vi "硬件定时参数设置.vi"(11 "硬件定时配置输入":T1) -> (3 "硬件定时配置输出":u32[](array[numeric]))   [LabVIEW 2012]
uses:
  u32-u8s.vi
  u16-u8s.vi
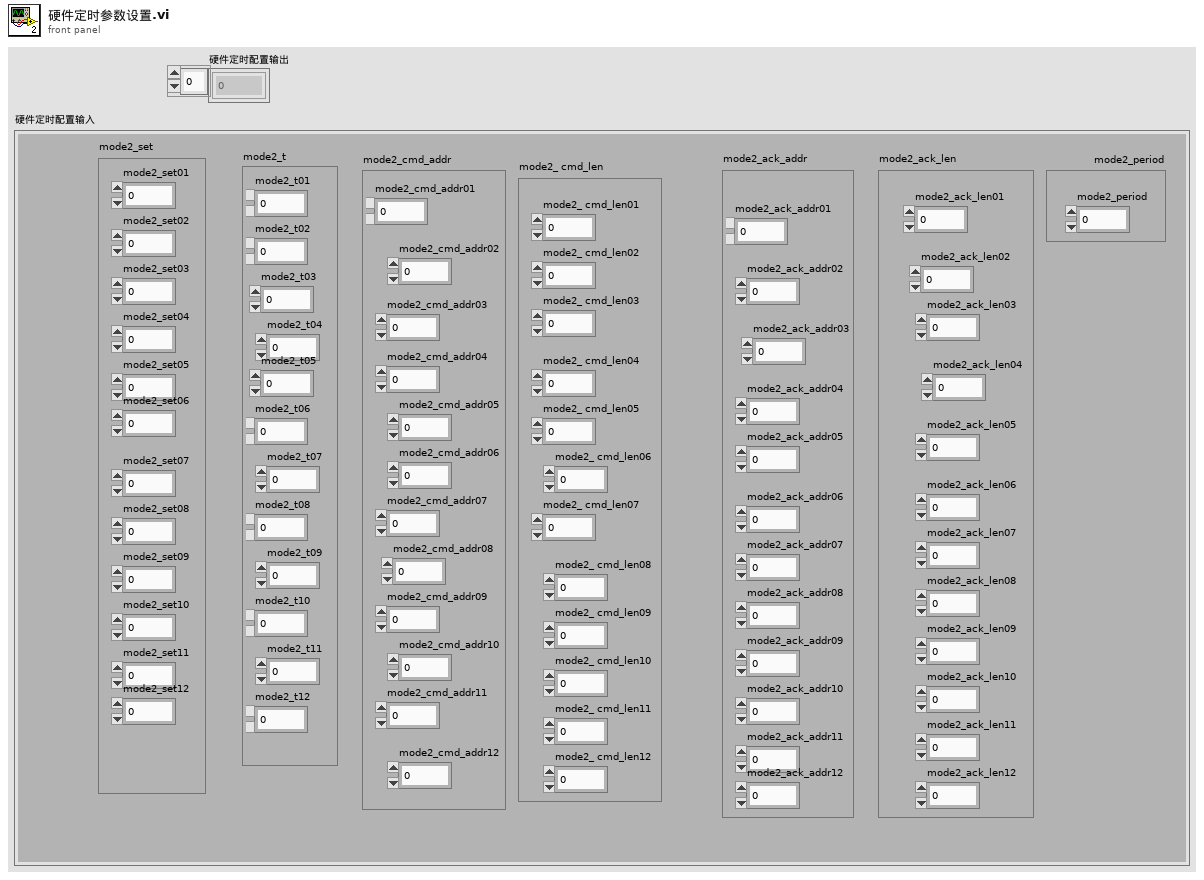
[diagram p1: front panel]
types:
  T1 = cluster{"mode2_set":cluster{"mode2_set01":u8, "mode2_set02":u8, "mode2_set03":u8, "mode2_set04":u8, "mode2_set05":u8, "mode2_set06":u8, "mode2_set07":u8, "mode2_set08":u8, "mode2_set09":u8, "mode2_set10":u8, "mode2_set11":u8, "mode2_set12":u8}, "mode2_t":cluster{"mode2_t01":u16, "mode2_t02":u16, "mode2_t03":u16, "mode2_t04":u16, "mode2_t05":u16, "mode2_t06":u16, "mode2_t07":u16, "mode2_t08":u16, "mode2_t09":u16, "mode2_t10":u16, "mode2_t11":u16, "mode2_t12":u16}, "mode2_cmd_addr":cluster{"mode2_cmd_addr01":u16, "mode2_cmd_addr02":u16, "mode2_cmd_addr03":u16, "mode2_cmd_addr04":u16, "mode2_cmd_addr05":u16, "mode2_cmd_addr06":u16, "mode2_cmd_addr07":u16, "mode2_cmd_addr08":u16, "mode2_cmd_addr09":u16, "mode2_cmd_addr10":u16, "mode2_cmd_addr11":u16, "mode2_cmd_addr12":u16}, "mode2_ cmd_len":cluster{"mode2_ cmd_len01":u16, "mode2_ cmd_len02":u16, "mode2_ cmd_len03":u16, "mode2_ cmd_len04":u16, "mode2_ cmd_len05":u16, "mode2_ cmd_len06":u16, "mode2_ cmd_len07":u16, "mode2_ cmd_len08":u16, "mode2_ cmd_len09":u16, "mode2_ cmd_len10":u16, "mode2_ cmd_len11":u16, "mode2_ cmd_len12":u16}, "mode2_ack_addr":cluster{"mode2_ack_addr01":u16, "mode2_ack_addr02":u16, "mode2_ack_addr03":u16, "mode2_ack_addr04":u16, "mode2_ack_addr05":u16, "mode2_ack_addr06":u16, "mode2_ack_addr07":u16, "mode2_ack_addr08":u16, "mode2_ack_addr09":u16, "mode2_ack_addr10":u16, "mode2_ack_addr11":u16, "mode2_ack_addr12":u16}, "mode2_ack_len":cluster{"mode2_ack_len01":u16, "mode2_ack_len02":u16, "mode2_ack_len03":u16, "mode2_ack_len04":u16, "mode2_ack_len05":u16, "mode2_ack_len06":u16, "mode2_ack_len07":u16, "mode2_ack_len08":u16, "mode2_ack_len09":u16, "mode2_ack_len10":u16, "mode2_ack_len11":u16, "mode2_ack_len12":u16}, "mode2_period":cluster{"mode2_period":u32}}
  T2 = cluster{"mode2_set01":u8, "mode2_set02":u8, "mode2_set03":u8, "mode2_set04":u8, "mode2_set05":u8, "mode2_set06":u8, "mode2_set07":u8, "mode2_set08":u8, "mode2_set09":u8, "mode2_set10":u8, "mode2_set11":u8, "mode2_set12":u8}
  T3 = cluster{"mode2_t01":u16, "mode2_t02":u16, "mode2_t03":u16, "mode2_t04":u16, "mode2_t05":u16, "mode2_t06":u16, "mode2_t07":u16, "mode2_t08":u16, "mode2_t09":u16, "mode2_t10":u16, "mode2_t11":u16, "mode2_t12":u16}
  T4 = cluster{"mode2_cmd_addr01":u16, "mode2_cmd_addr02":u16, "mode2_cmd_addr03":u16, "mode2_cmd_addr04":u16, "mode2_cmd_addr05":u16, "mode2_cmd_addr06":u16, "mode2_cmd_addr07":u16, "mode2_cmd_addr08":u16, "mode2_cmd_addr09":u16, "mode2_cmd_addr10":u16, "mode2_cmd_addr11":u16, "mode2_cmd_addr12":u16}
  T5 = cluster{"mode2_ cmd_len01":u16, "mode2_ cmd_len02":u16, "mode2_ cmd_len03":u16, "mode2_ cmd_len04":u16, "mode2_ cmd_len05":u16, "mode2_ cmd_len06":u16, "mode2_ cmd_len07":u16, "mode2_ cmd_len08":u16, "mode2_ cmd_len09":u16, "mode2_ cmd_len10":u16, "mode2_ cmd_len11":u16, "mode2_ cmd_len12":u16}
  T6 = cluster{"mode2_ack_addr01":u16, "mode2_ack_addr02":u16, "mode2_ack_addr03":u16, "mode2_ack_addr04":u16, "mode2_ack_addr05":u16, "mode2_ack_addr06":u16, "mode2_ack_addr07":u16, "mode2_ack_addr08":u16, "mode2_ack_addr09":u16, "mode2_ack_addr10":u16, "mode2_ack_addr11":u16, "mode2_ack_addr12":u16}
  T7 = cluster{"mode2_ack_len01":u16, "mode2_ack_len02":u16, "mode2_ack_len03":u16, "mode2_ack_len04":u16, "mode2_ack_len05":u16, "mode2_ack_len06":u16, "mode2_ack_len07":u16, "mode2_ack_len08":u16, "mode2_ack_len09":u16, "mode2_ack_len10":u16, "mode2_ack_len11":u16, "mode2_ack_len12":u16}
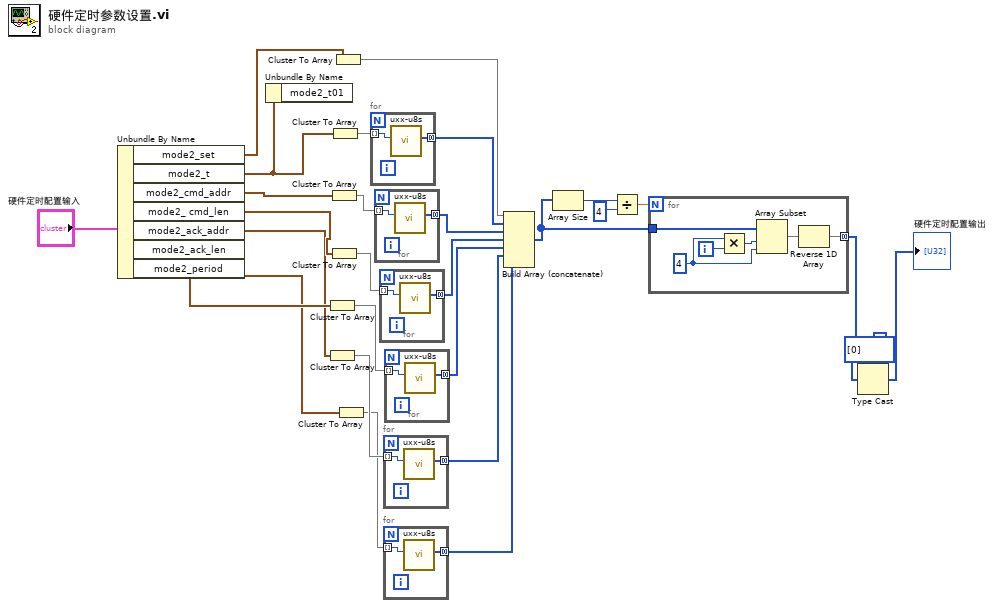
[diagram p0: block diagram]
diagram:
  n1 = Unbundle By Name("硬件定时配置输入") -> ("mode2_set"=w2:T2, "mode2_t"=w1:T3, "mode2_cmd_addr"=w26:T4, "mode2_ cmd_len"=w25:T5, "mode2_ack_addr"=w23:T6, "mode2_ack_len"=w22:T7, "mode2_period"=w24:cluster{"mode2_period":u32})
  n2 = Unbundle By Name(w1) -> ()  [unwired: 1 out]
  n3 = Cluster To Array(cluster=w24) -> (array=w15:u32[])
  n4 = Cluster To Array(cluster=w23) -> (array=w13:u16[])
  n5 = Cluster To Array(cluster=w26) -> (array=w19:u16[])
  n6 = Cluster To Array(cluster=w25) -> (array=w17:u16[])
  n7 = Cluster To Array(cluster=w1) -> (array=w21:u16[])
  n8 = Cluster To Array(cluster=w2) -> (array=w28:u8[])
  n9 = Cluster To Array(cluster=w22) -> (array=w11:u16[])
  n10 = for {
    tunnel: w21 -> [w30] mode=indexing
    tunnel: [w29] -> w20 mode=concatenating
    n11 = call-poly "uxx-u8s.vi"("数值"=w30) -> ("反转的数组"=w29:u8[])  [unwired: 10 in]
  }
  n12 = for {
    tunnel: w19 -> [w32] mode=indexing
    tunnel: [w31] -> w18 mode=concatenating
    n13 = call-poly "uxx-u8s.vi"("数值"=w32) -> ("反转的数组"=w31:u8[])  [unwired: 10 in]
  }
  n14 = for {
    tunnel: w17 -> [w34] mode=indexing
    tunnel: [w33] -> w16 mode=concatenating
    n15 = call-poly "uxx-u8s.vi"("数值"=w34) -> ("反转的数组"=w33:u8[])  [unwired: 10 in]
  }
  n16 = for {
    tunnel: w13 -> [w36] mode=indexing
    tunnel: [w35] -> w12 mode=concatenating
    n17 = call-poly "uxx-u8s.vi"("数值"=w36) -> ("反转的数组"=w35:u8[])  [unwired: 10 in]
  }
  n18 = for {
    tunnel: w11 -> [w38] mode=indexing
    tunnel: [w37] -> w10 mode=concatenating
    n19 = call-poly "uxx-u8s.vi"("数值"=w38) -> ("反转的数组"=w37:u8[])  [unwired: 10 in]
  }
  n20 = for {
    tunnel: w15 -> [w40] mode=indexing
    tunnel: [w39] -> w14 mode=concatenating
    n21 = call-poly "uxx-u8s.vi"("数值"=w40) -> ("反转的数组"=w39:u8[])  [unwired: 10 in]
  }
  n22 = Build Array (concatenate)(w28, w20, w18, w16, w14, w12, w10) -> (w6:u8[])
  n23 = Array Size(array=w6) -> (size(s)=w9:i32)
  n24 = Divide(x=w9, y=4) -> (x/y=w7:dbl)
  n25 = for {
    N: w7 -> [_]
    tunnel: w6 -> [w46]
    tunnel: [w41] -> w4 mode=concatenating
    i -> [w45]
    w43 = 4 ("x")
    n26 = Multiply(x=w43, y=w45) -> (x*y=w44:i32)
    n27 = Array Subset(array=w46, index=w44, length=w43) -> (w42:u8[])
    n28 = Reverse 1D Array(array=w42) -> (reversed array=w41:u8[])
  }
  n29 = Type Cast(type=u32[] [0], x=w4) -> (*(type *) &x=→"硬件定时配置输出":u32[])
